vi "Core Actor - INIT - External Queues_Notifiers.vi"(8 "error in (no error)":errorcluster, 11 "Parent_Class in":refnum<class "Message_Distributor_Class.lvclass">) -> (0 "error out":errorcluster, 3 "Parent_Class out":refnum<class "Message_Distributor_Class.lvclass">)   [LabVIEW 2023, in "Actor_Message_Distributor.lvlib" / "Message_Distributor_Class.lvclass"]
uses:
  Message_Distributor_Class.lvclass
  Message_Distributor_Class.lvclass/Message_Distributor_Class.ctl
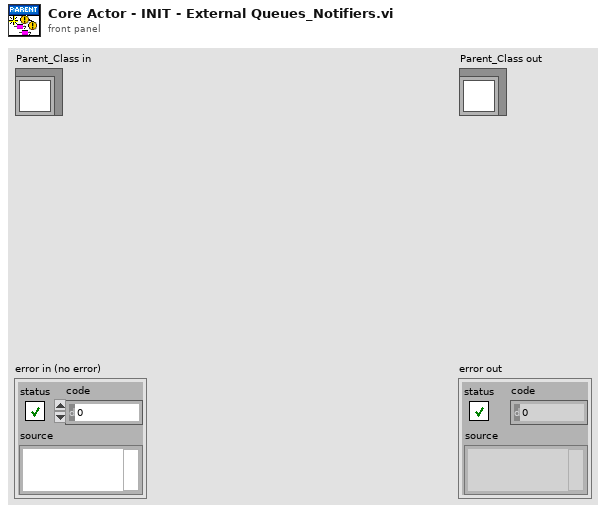
[diagram p1: front panel]
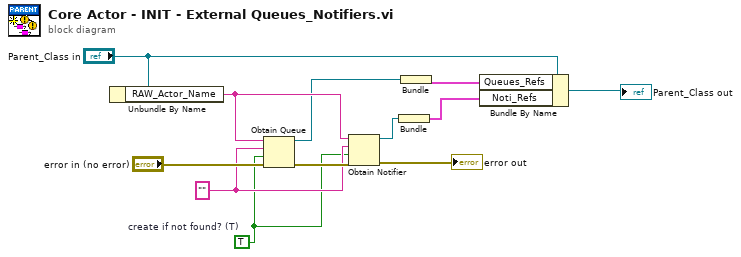
[diagram p0: block diagram]
diagram:
  w8 = TRUE  # create if not found? (T)
  w9 = ""
  n1 = Unbundle By Name("Parent_Class in") -> ("RAW_Actor_Name"=w10:string)
  n2 = Obtain Queue(name (unnamed)=w10, element data type=w9, create if not found? (T)=w8, error in (no error)="error in (no error)") -> (queue out=w4:refnum<queue>, error out=w11:errorcluster)  [unwired: 1 in, 1 out]
  n3 = Obtain Notifier(name (unnamed)=w10, notification data type=w9, create if not found? (T)=w8, error in (no error)=w11) -> (notifier out=w2:refnum<notifier>, error out=→"error out":errorcluster)  [unwired: 1 out]
  n4 = Bundle("notifier out"=w2) -> (w1:cluster{"notifier out":refnum<notifier>})  [unwired: 1 in]
  n5 = Bundle("queue out"=w4) -> (w3:cluster{"queue out":refnum<queue>})  [unwired: 1 in]
  n6 = Bundle By Name(cluster="Parent_Class in", "Queues_Refs"=w3, "Noti_Refs"=w1) -> (→"Parent_Class out":refnum<class "Message_Distributor_Class.lvclass">)
